vi "Draw Triangle.vi"(6 "Pen":T1={"Width"=1, "Style"=enum."Solid"}, 8 "Point 3":T2, 9 "Point 2":T2, 10 "Point 1":T2, 11 "Picture in":picture) -> (3 "Picture out":picture)   [LabVIEW 2020]
uses:
  Controls/Point 2D.ctl
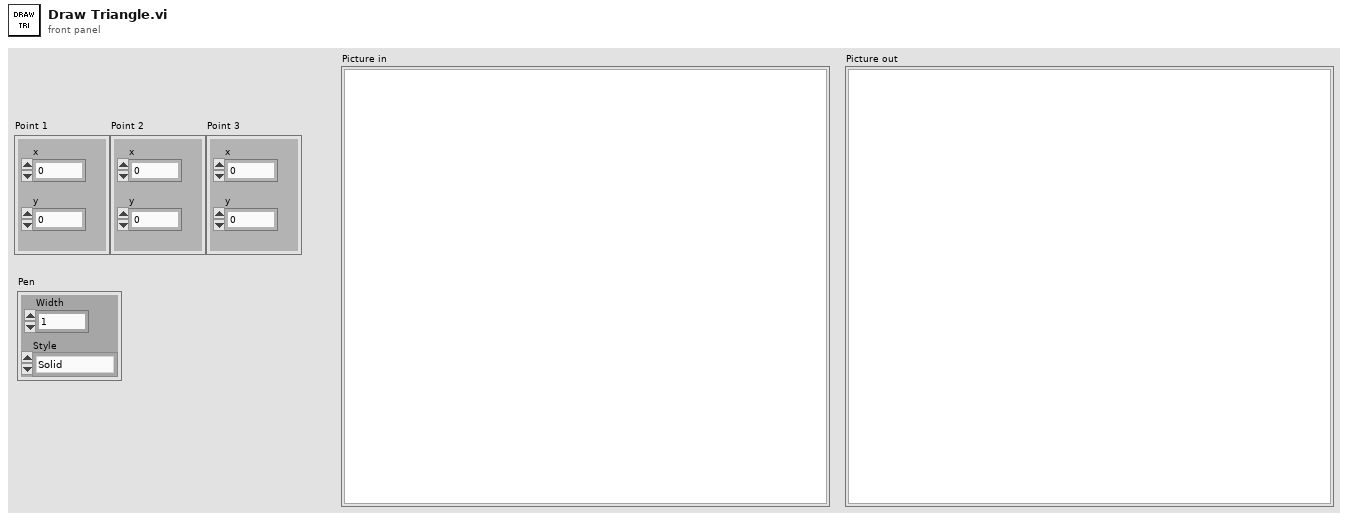
[diagram p1: front panel]
types:
  T1 = cluster{"Width":u16, "Style":enum32{"Solid", "Dash", "Dot", "DashDot", "DashDotDot"}}
  T2 = typedef "Point 2D.ctl" = cluster{"x":sgl, "y":sgl}
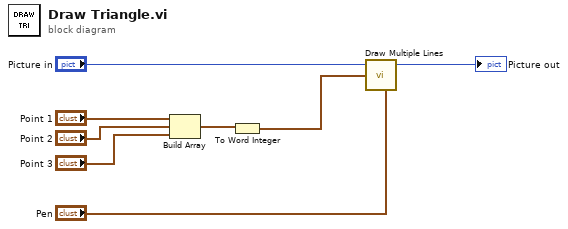
[diagram p0: block diagram]
diagram:
  n1 = Build Array("Point 1", "Point 2", "Point 3") -> (w5:T2[])
  n2 = To Word Integer(number=w5) -> (16bit integer=w4:cluster{"x":i16, "y":i16}[])
  n3 = call <vilib>:"Draw Multiple Lines.vi"("picture"="Picture in", "line endpoints"=w4, "pen"="Pen") -> ("new picture"=→"Picture out":picture)  [unwired: 6 in]
